vi "IMAQ subtract background.vi"(7 "FakeCamera in":refnum<class "Point Grey Camera.lvclass">, 8 "error in (no error)":errorcluster, 11 "Image in":T1) -> (0 "error out":errorcluster, 1 "Intensity Graph":u16[][](graph), 2 "Line Graph 2":cluster{"x0":sgl, "dx":sgl, "Pixels Line":sgl[]} {"dx" format="%.2f"; "x0" format="%.2f"}, 3 "Refnum out":T1, 4 "Line Graph":cluster{"x0":sgl, "dx":sgl, "Pixels Line":sgl[]} {"dx" format="%.2f"; "x0" format="%.2f"}, 5 "FakeCamera out":refnum<class "Point Grey Camera.lvclass">)   [LabVIEW 2020, in "Point Grey Camera.lvclass"]
uses:
  Point Grey Camera.lvclass
  <vilib>/vision/Image Controls.llb/IMAQ Image.ctl
  Point Grey Camera.lvclass/Point Grey Camera.ctl
  <vilib>/Analysis/1siggen.llb/Ramp Pattern by Samples.vi
  <userlib>/_OpenG.lib/file/file.llb/File Exists - Scalar__ogtk.vi
  <vilib>/vision/NI_Vision_Development_Module.lvlib
  <vilib>/Analysis/NI_AALBase.lvlib
panel:
  out "create BG":u32
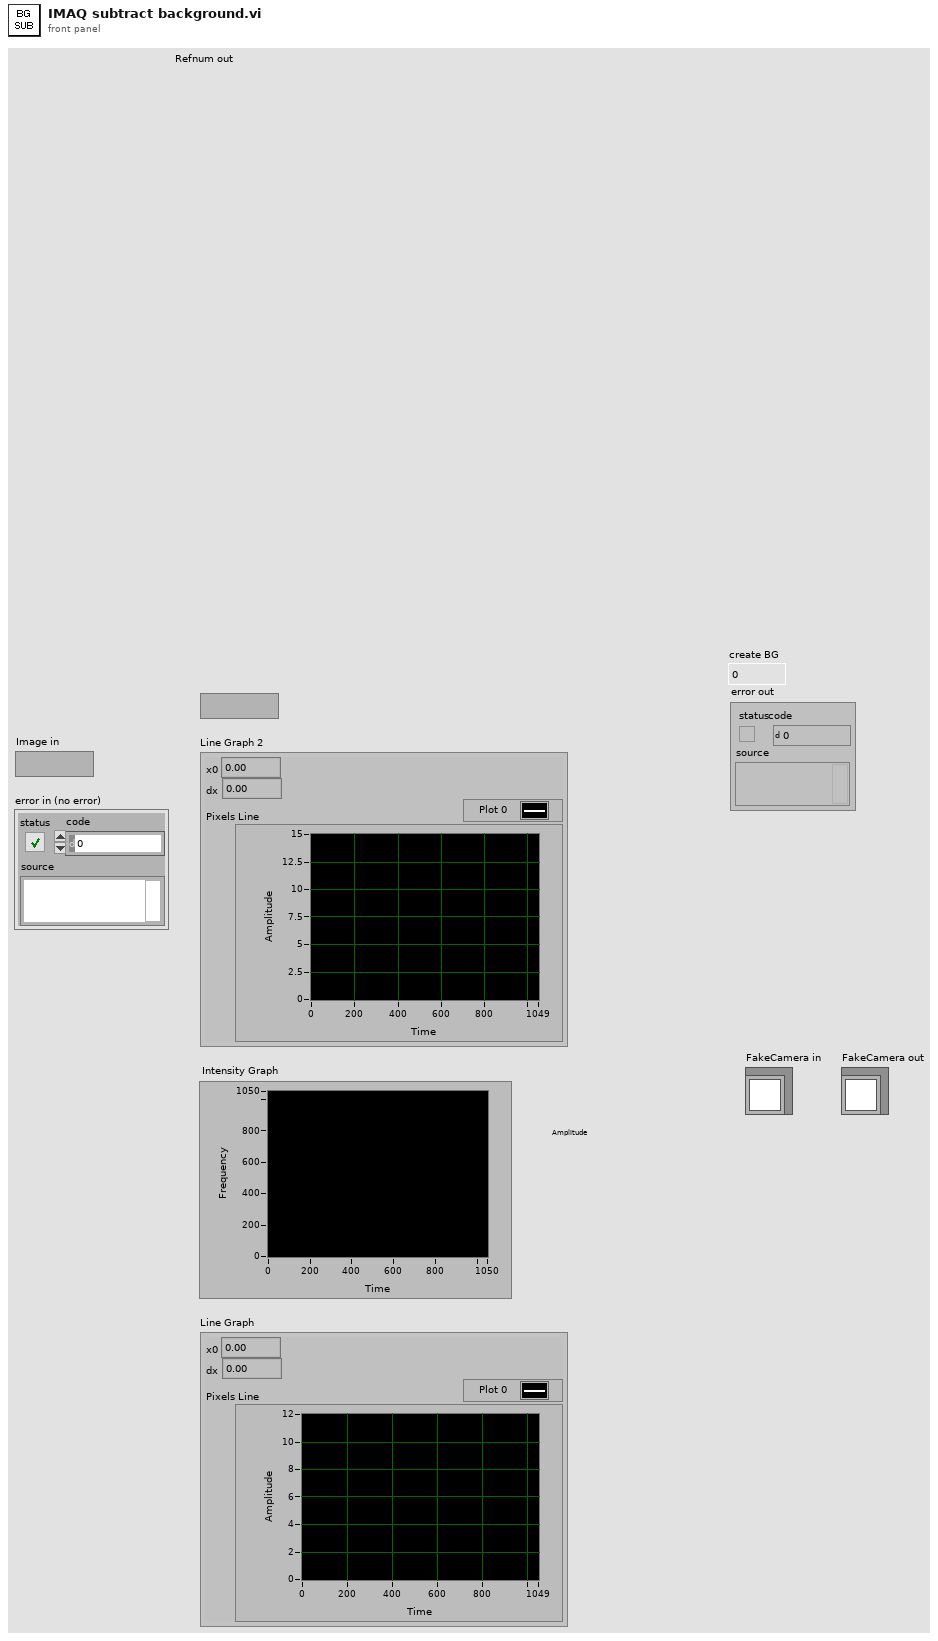
[diagram p1: front panel]
types:
  T1 = typedef "IMAQ Image.ctl" = refnum<image>
  T2 = cluster{"X Size":i32, "Y Size":i32, "% Tolerance":i32}
  T3 = typedef "ROI Descriptor" = cluster{"Global Rectangle":i32[], "Contours":cluster{"ID":enum32{"External", "Internal"}, "Type":u32, "Coordinates":i32[]}[]}
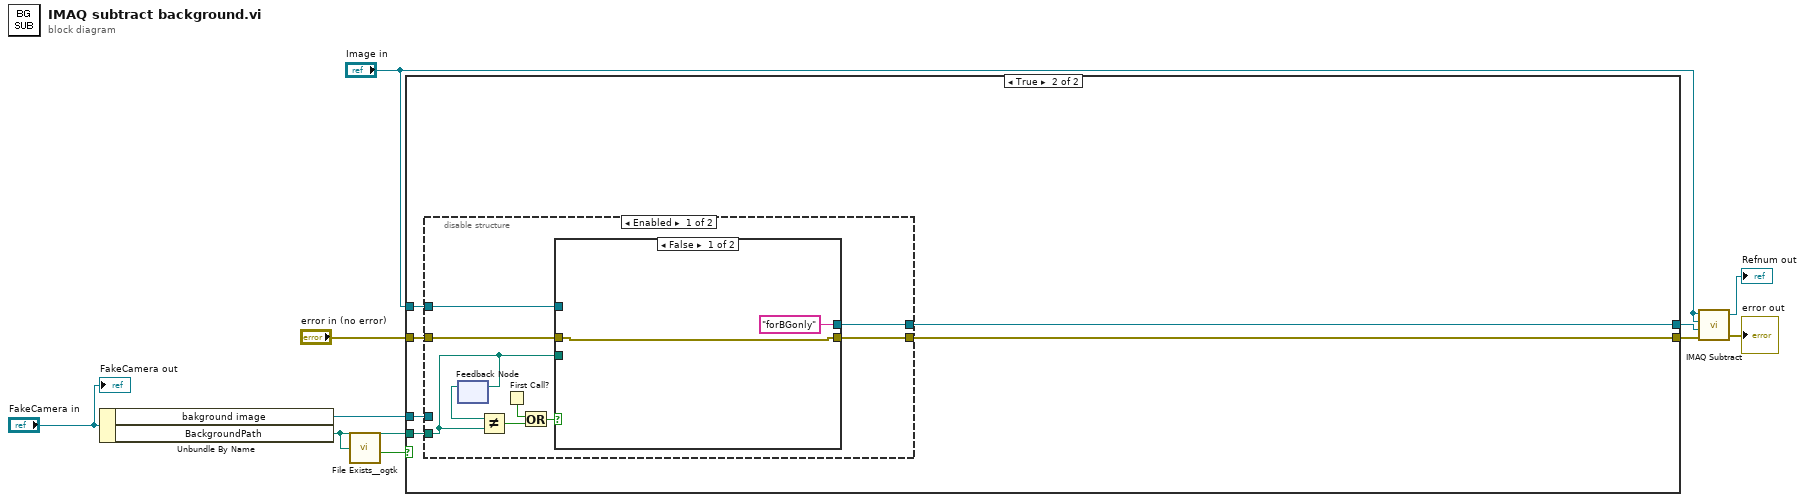
[diagram p0: block diagram]
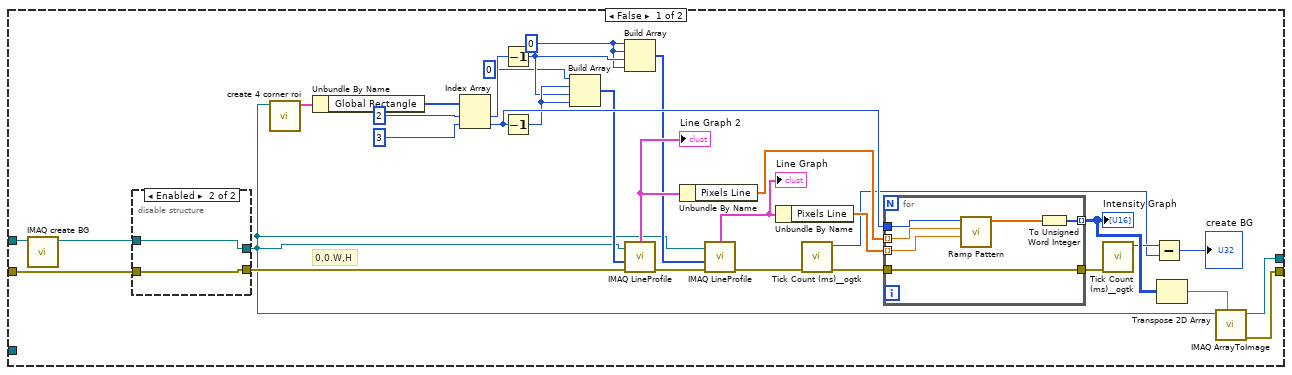
[diagram p2: hidden frame]
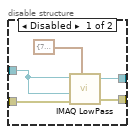
[diagram p3: hidden frame]
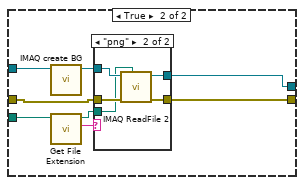
[diagram p4: hidden frame]
diagram:
  n1 = Unbundle By Name("FakeCamera in") -> ("bakground image"=w1:T1, "BackgroundPath"=w4:path)
  n2 = call-poly <userlib>:"File Exists__ogtk.vi"("file path"=w4) -> ("exists"=w6:bool)  [unwired: 6 in, 1 out]
  n3 = case shown="True" w6 {
    tunnel: "error in (no error)" -> [w41 w58]
    tunnel: [w40 w57] -> w8
    tunnel: [w37 w59] -> w7
    tunnel: "Image in" -> [w12 w61]
    tunnel: w4 -> [_ w60]
    tunnel: w1 -> [_ w56]
    frame False {
      w29 = 0 ("element")
      # "0,0.W,H"
      n4 = call "IMAQ create BG.vi"("Refnum in"=w12) -> ("Refnum out"=w11:T1)  [unwired: 10 in]
      n5 = disable-structure shown="Enabled" {
        disable-tunnel: w11 -> [w47 w49]
        disable-tunnel: w41 -> [w46 w48]
        disable-tunnel: [w45 w48] -> w38
        disable-tunnel: [w43 w49] -> w19
        frame Disabled {
          n6 = call "IMAQ LowPass"("Image Src"=w47, "Size & Tolerance"=T2 {"X Size"=7, "Y Size"=7, "% Tolerance"=10}, "Image Dst"=w47, "error in (no error)"=w46) -> ("Image Dst Out"=w43:T1, "error out"=w45:errorcluster)  [unwired: 3 in]
        }
        frame Enabled {
        }
      }
      n7 = call "create 4 corner roi.vi"("Refnum in"=w19) -> ("ROI Descriptor"=w42:T3)  [unwired: 9 in, 1 out]
      n8 = Unbundle By Name(w42) -> ("Global Rectangle"=w20:i32[])
      n9 = Index Array(array=w20, index #1=2 ("index"), index #2=3 ("index")) -> (element #1=w32:i32, element #2=w34:i32)
      n10 = Decrement(x=w32) -> (x-1=w31:i32)
      n11 = Decrement(x=w34) -> (x-1=w33:i32)
      n12 = Build Array(0 ("element"), w33, w31, w33) -> (w24:i32[])
      n13 = Build Array(w29, w29, w31, w29) -> (w23:i32[])
      n14 = call "IMAQ LineProfile"("error in (no error)"=w38, "Line Coordinates"=w24, "Image"=w19) -> ("error out"=w39:errorcluster, "Line Graph"=w26:cluster{"x0":sgl, "dx":sgl, "Pixels Line":sgl[]})  [unwired: 2 in, 2 out]
      "Line Graph 2" <- w26
      n15 = Unbundle By Name(w26) -> ("Pixels Line"=w28:sgl[])
      n16 = call "IMAQ LineProfile"("error in (no error)"=w39, "Line Coordinates"=w23, "Image"=w19) -> ("error out"=w18:errorcluster, "Line Graph"=w25:cluster{"x0":sgl, "dx":sgl, "Pixels Line":sgl[]})  [unwired: 2 in, 2 out]
      "Line Graph" <- w25
      n17 = Unbundle By Name(w25) -> ("Pixels Line"=w27:sgl[])
      n18 = call <userlib>:"Tick Count (ms)__ogtk.vi"("error in (no error)"=w18) -> ("error out"=w17:errorcluster, "millisecond timer value"=w14:u32)  [unwired: 9 in]
      n19 = for {
        tunnel: w27 -> [w53] mode=indexing
        tunnel: w28 -> [w54] mode=indexing
        tunnel: w34 -> [w55]
        tunnel: [w51] -> w35 mode=indexing
        tunnel: w17 -> [w50]
        tunnel: [w50] -> w16
        n20 = call-poly <vilib>:"Ramp Pattern.vi"("start"=w53, "end"=w54, "samples"=w55) -> ("Ramp Pattern"=w52:dbl[])  [unwired: 7 in, 1 out]
        n21 = To Unsigned Word Integer(number=w52) -> (unsigned 16bit integer=w51:u16[])
      }
      "Intensity Graph" <- w35
      n22 = call <userlib>:"Tick Count (ms)__ogtk.vi"("error in (no error)"=w16) -> ("millisecond timer value"=w15:u32)  [unwired: 9 in, 1 out]
      n23 = Subtract(x=w15, y=w14) -> (x-y=→"create BG":u32)
      n24 = Transpose 2D Array(2D array=w35) -> (transposed array=w36:u16[][])
      n25 = call "IMAQ ArrayToImage"("Image Pixels (U16)"=w36, "Image"=w19) -> ("error out"=w40:errorcluster, "Image Out"=w37:T1)  [unwired: 8 in]
    }
    frame True {
      n26 = disable-structure shown="Enabled" {
        disable-tunnel: w61 -> [w70 _]
        disable-tunnel: w60 -> [w65 _]
        disable-tunnel: [w69 w88] -> w59
        disable-tunnel: w58 -> [w68 _]
        disable-tunnel: [w67 _] -> w57
        disable-tunnel: w56 -> [_ w88]
        frame Enabled {
          n27 = feedback-in #1(w65) -> ()
          n28 = feedback #1() -> (w66:path)  [unwired: 1 in]
          n29 = Not Equal?(x=w66, y=w65) -> (x != y?=w63:bool)
          n30 = First Call?() -> (First Call?: T/F=w64:bool)
          n31 = Or(x=w64, y=w63) -> (x .or. y?=w62:bool)
          n32 = case shown="False" w62 {
            tunnel: w70 -> [_ w80]
            tunnel: w65 -> [_ w79]
            tunnel: ["forBGonly" ("Image Name") w76] -> w69
            tunnel: w68 -> [w72 w75]
            tunnel: [w72 w74] -> w67
            frame False {
            }
            frame True {
              n33 = call "IMAQ create BG.vi"("Refnum in"=w80) -> ("Refnum out"=w77:T1)  [unwired: 10 in]
              n34 = call <vilib>:"Get File Extension.vi"("file"=w79) -> ("lowercase file extension"=w78:string, "dup file"=w73:path)  [unwired: 6 in, 3 out]
              n35 = case shown="\"png\"" w78 {
                tunnel: w77 -> [w82 w87]
                tunnel: [w82 w86] -> w76
                tunnel: w75 -> [w81 w85]
                tunnel: [w81 w84] -> w74
                tunnel: w73 -> [_ w83]
                frame "False", Default {
                }
                frame "png" {
                  n36 = call "IMAQ ReadFile 2"("File Path"=w83, "error in (no error)"=w85, "Image"=w87) -> ("error out"=w84:errorcluster, "Image Out"=w86:T1)  [unwired: 4 in, 3 out]
                }
              }
            }
          }
        }
        frame Disabled {
        }
      }
    }
  }
  n37 = call "IMAQ Subtract"("Image Src A"="Image in", "Image Dst"="Image in", "Image Src B"=w7, "error in (no error)"=w8) -> ("Image Dst Out"=→"Refnum out":T1, "error out"=→"error out":errorcluster)  [unwired: 3 in]
  "FakeCamera out" <- "FakeCamera in"
